vi "cpx print test.vi"() -> ()   [LabVIEW 2020]
panel:
  out "decimal integer string":string
  in  "Complex":T1
types:
  T1 = cluster{"Real":fxp<+/-,32,11>, "Imag":fxp<+/-,32,11>}
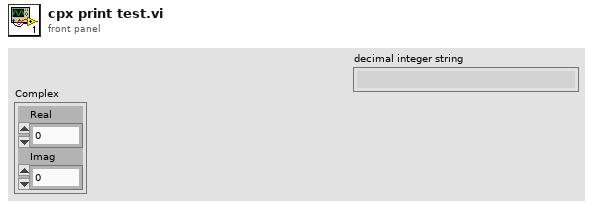
[diagram p1: front panel]
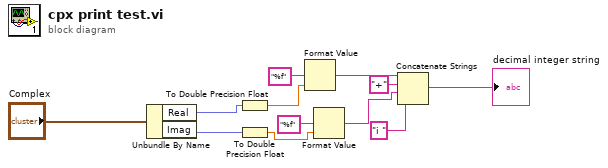
[diagram p0: block diagram]
diagram:
  n1 = Unbundle By Name("Complex") -> ("Real"=w2:fxp<+/-,32,11>, "Imag"=w1:fxp<+/-,32,11>)
  n2 = To Double Precision Float(number=w2) -> (double precision float=w10:dbl)
  n3 = To Double Precision Float(number=w1) -> (double precision float=w8:dbl)
  n4 = Format Value(format string="%f", value (0)=w10) -> (output string=w7:string)  [unwired: 1 in]
  n5 = Format Value(format string="%f", value (0)=w8) -> (output string=w5:string)  [unwired: 1 in]
  n6 = Concatenate Strings(w7, "+" ("string"), w5, "i " ("string")) -> (→"decimal integer string":string)
